vi "InfoRead4.vi"(4 "data info template":refnum<vi>, 5 "source path":string) -> (2 "data from *.info.txt":T1)   [LabVIEW 2014]
uses:
  <vilib>/Utility/file.llb/Read From Spreadsheet File (string).vi
panel:
  # "0 - aplly *.info.txt\n1 - Continue and enter the data manually\n2 - Cancel and correct the *.info.txt"
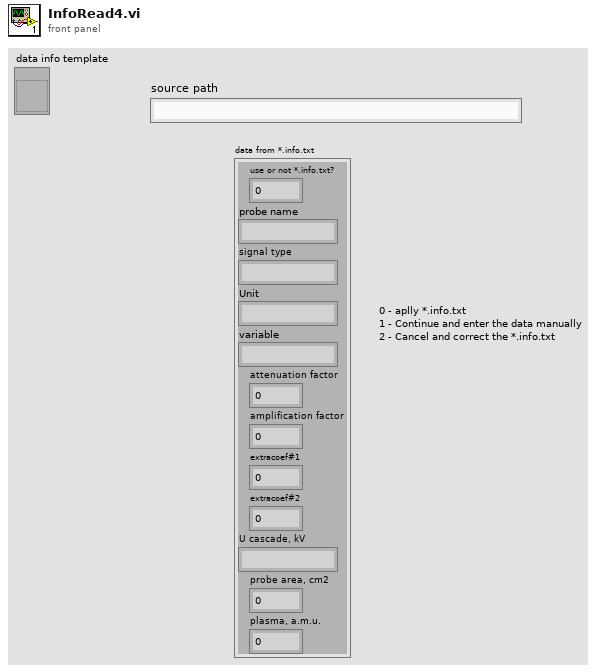
[diagram p1: front panel]
types:
  T1 = cluster{"use or not *.info.txt?":i16, "probe name":string, "signal type":string, "Unit":string, "variable":string, "attenuation factor":dbl, "amplification factor":dbl, "extracoef#1":dbl, "extracoef#2":dbl, "U cascade, kV":string, "probe area, cm2":dbl, "plasma, a.m.u.":dbl}
  T2 = cluster{"data path":string, "ADCintercadr_s":dbl, "data info":cluster{"use or not *.info.txt?":i16, "probe name":string, "signal type":string, "Unit":string, "variable":string, "attenuation factor":dbl, "amplification factor":dbl, "extracoef#1":dbl, "extracoef#2":dbl, "U cascade, kV":string, "probe area, cm2":dbl, "plasma, a.m.u.":dbl}, "channel_name":string, "channels_in_file":i32, "LastModified":string}
  T3 = enum16{"Left Button", "Center Button", "Right Button", "Window Close"}
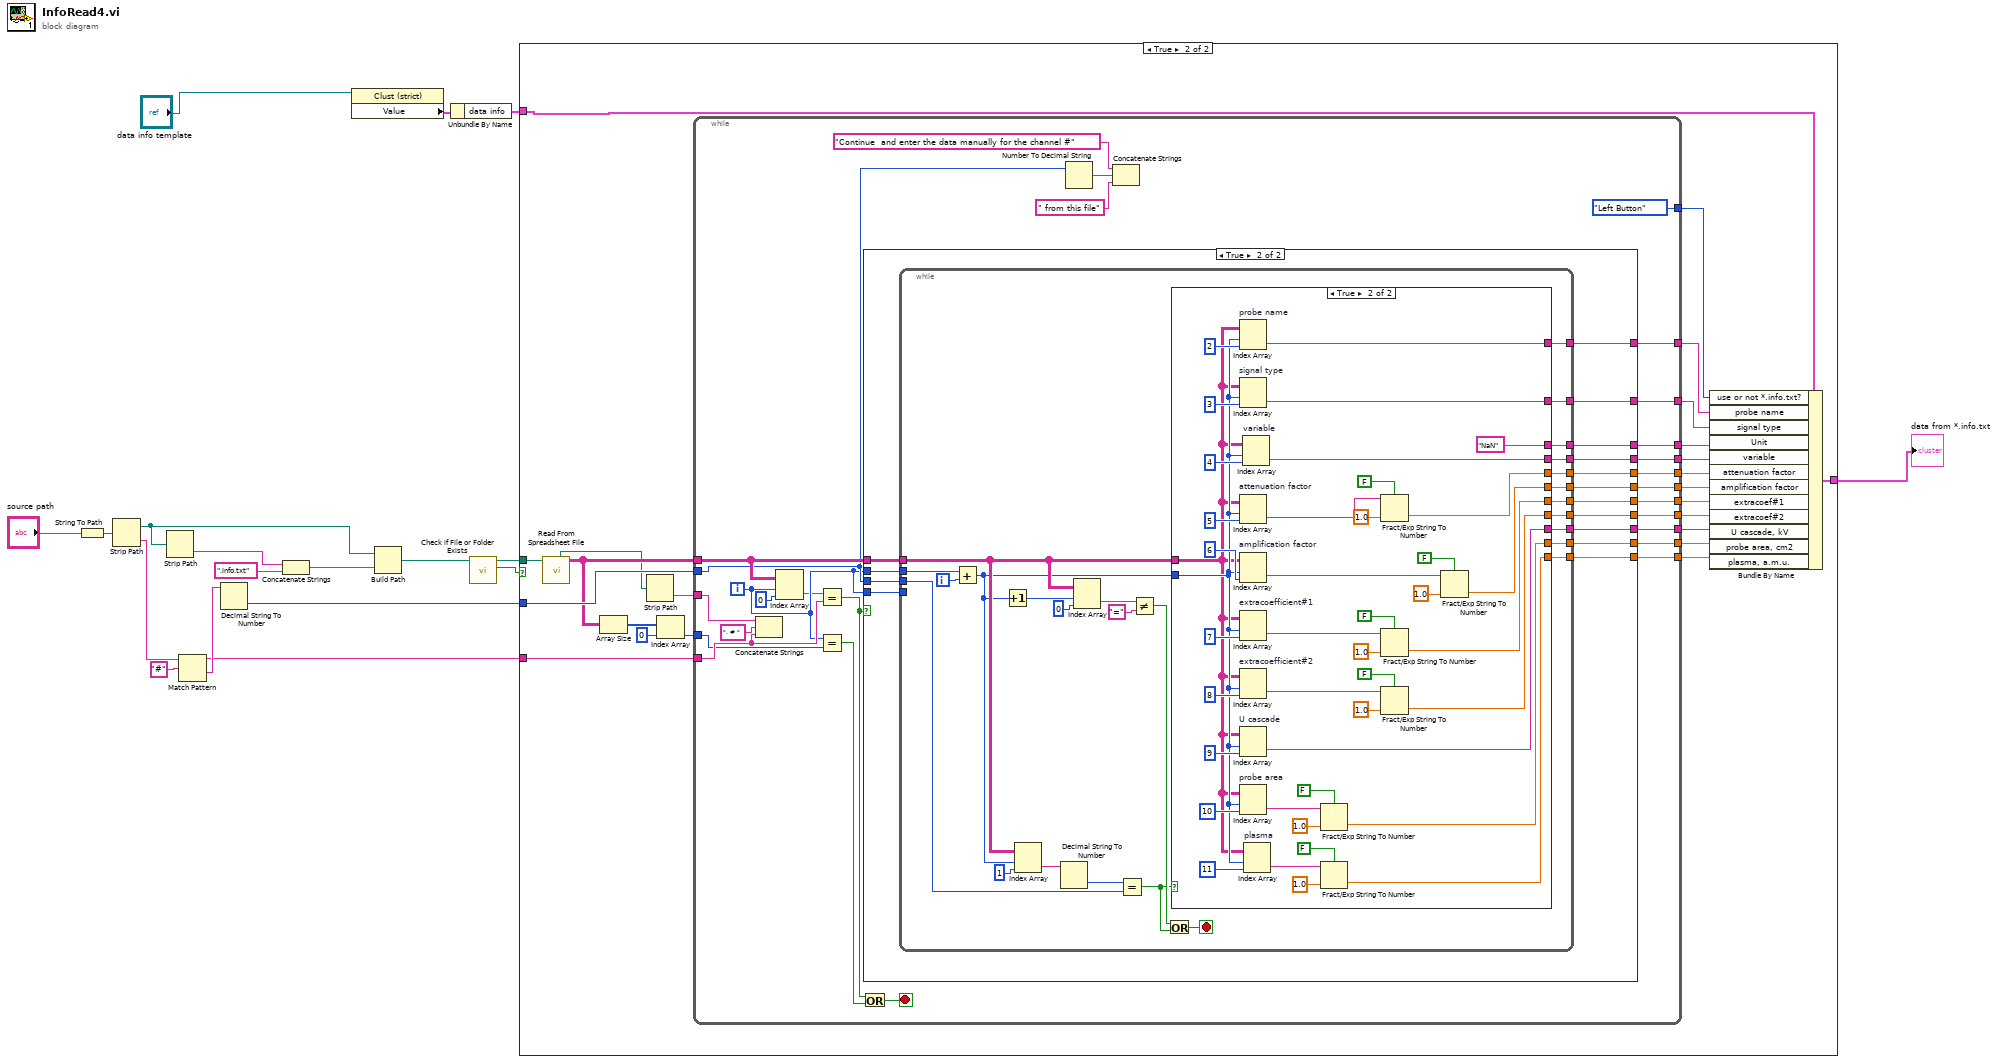
[diagram p0: block diagram]
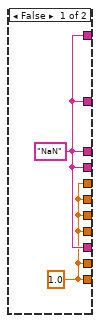
[diagram p3: hidden frame]
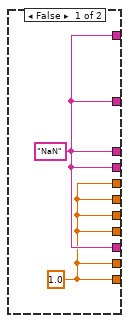
[diagram p4: hidden frame]
diagram:
  n1 = String To Path(string="source path") -> (path=w13:path)
  n2 = Strip Path(path=w13) -> (stripped path=w7:path, name=w17:string)
  n3 = Strip Path(path=w7) -> (name=w6:string)  [unwired: 1 out]
  n4 = Match Pattern(string=w17, regular expression="#") -> (before substring=w12:string, after substring=w15:string)  [unwired: 1 in, 2 out]
  n5 = Decimal String To Number(string=w15) -> (number=w14:i32)  [unwired: 2 in, 1 out]
  n6 = Concatenate Strings(w6, ".info.txt" ("string")) -> (w10:string)
  n7 = property class="Clust (strict)"(reference="data info template") -> ("Value"=w4:T2)  [unwired: 1 in, 2 out]
  n8 = Build Path(base path=w7, name or relative path=w10) -> (appended path=w9:path)
  n9 = Unbundle By Name(w4) -> ("data info"=w3:T1)
  n10 = call <vilib>:"Check if File or Folder Exists.vi"("path"=w9) -> ("file or folder exists?"=w5:bool, "dup path"=w8:path)  [unwired: 8 in, 1 out]
  n11 = case shown="True" w5 {
    tunnel: w14 -> [_ w39]
    tunnel: w12 -> [_ w38]
    tunnel: w8 -> [_ w36]
    tunnel: [w19 w20] -> w2
    tunnel: w3 -> [w19 w21]
    frame False {
    }
    frame True {
      n12 = call-poly <vilib>:"Read From Spreadsheet File.vi"("file path (dialog if empty)"=w36) -> ("all rows"=w37:string[][], "new file path (Not A Path if cancelled)"=w35:path)  [unwired: 6 in, 3 out]
      n13 = Array Size(array=w37) -> (size(s)=w41:i32[])
      n14 = Strip Path(path=w35) -> (name=w40:string)  [unwired: 1 out]
      n15 = Index Array(array=w41, index=0) -> (element=w34:i32)
      n16 = while {
        tunnel: w37 -> [w65]
        tunnel: [T3."Left Button" ("Which Button?")] -> w33
        tunnel: w39 -> [w59]
        tunnel: w40 -> [w61]
        tunnel: w38 -> [w58]
        tunnel: w34 -> [w57]
        tunnel: [w56] -> w32
        tunnel: [w55] -> w31
        tunnel: [w54] -> w30
        tunnel: [w53] -> w29
        tunnel: [w52] -> w28
        tunnel: [w51] -> w27
        tunnel: [w50] -> w26
        tunnel: [w49] -> w25
        tunnel: [w48] -> w24
        tunnel: [w47] -> w23
        tunnel: [w46] -> w22
        i -> [w45]
        stop <- w68 stop-if-true
        n17 = Concatenate Strings(w61, ", # " ("string"), w58) -> ()  [unwired: 1 out]
        n18 = Index Array(array=w65, index (row)=w45, index (col)=0 ("disabled index (col)")) -> (element=w44:string)
        n19 = Equal?(x=w44, y=w58) -> (x = y?=w66:bool)
        n20 = Equal?(x=w45, y=w57) -> (x = y?=w67:bool)
        n21 = Or(x=w66, y=w67) -> (x .or. y?=w68:bool)
        n22 = case shown="True" w66 {
          tunnel: w65 -> [_ w73]
          tunnel: w59 -> [_ w86]
          tunnel: w45 -> [_ w85]
          tunnel: [w71 w83] -> w56
          tunnel: [w71 w82] -> w55
          tunnel: [w71 w84] -> w54
          tunnel: [w71 w81] -> w53
          tunnel: [w71 w76] -> w52
          tunnel: [w70 w80] -> w51
          tunnel: [w70 w79] -> w50
          tunnel: [w70 w78] -> w49
          tunnel: [w70 w77] -> w48
          tunnel: [w70 w75] -> w47
          tunnel: [w70 w74] -> w46
          tunnel: w45 -> [_ w72]
          frame False {
            w70 = 1.0
            w71 = "NaN" ("String")
          }
          frame True {
            n23 = while {
              tunnel: w86 -> [w112]
              tunnel: w85 -> [_]
              tunnel: [w111] -> w84
              tunnel: [w110] -> w83
              tunnel: [w109] -> w82
              tunnel: [w108] -> w81
              tunnel: [w107] -> w80
              tunnel: [w106] -> w79
              tunnel: [w105] -> w78
              tunnel: [w104] -> w77
              tunnel: [w103] -> w76
              tunnel: [w102] -> w75
              tunnel: [w101] -> w74
              tunnel: w73 -> [w94]
              tunnel: w72 -> [w98]
              i -> [w97]
              stop <- w89 stop-if-true
              n24 = Add(x=w98, y=w97) -> (x+y=w90:i32)
              n25 = Increment(x=w90) -> (x+1=w91:i32)
              n26 = Index Array(array=w94, index (row)=w90, index (col)=1 ("disabled index (col)")) -> (element=w99:string)
              n27 = Decimal String To Number(string=w99) -> (number=w100:i32)  [unwired: 2 in, 1 out]
              n28 = Index Array(array=w94, index (row)=w91, index (col)=0 ("disabled index (col)")) -> (element=w93:string)
              n29 = Equal?(x=w100, y=w112) -> (x = y?=w87:bool)
              n30 = Not Equal?(x=w93, y="=") -> (x != y?=w88:bool)
              n31 = Or(x=w88, y=w87) -> (x .or. y?=w89:bool)
              n32 = case shown="True" w87 {
                tunnel: [w114 "NaN"] -> w111
                tunnel: [w114 w130] -> w110
                tunnel: [w114 w129] -> w109
                tunnel: [w114 w128] -> w108
                tunnel: [w113 w127] -> w107
                tunnel: [w113 w126] -> w106
                tunnel: [w113 w125] -> w105
                tunnel: w90 -> [_ w123]
                tunnel: [w113 w119] -> w104
                tunnel: [w114 w118] -> w103
                tunnel: [w113 w117] -> w102
                tunnel: [w113 w116] -> w101
                tunnel: w94 -> [_ w115]
                frame False {
                  w113 = 1.0
                  w114 = "NaN"
                }
                frame True {
                  n33 = Index Array "probe name"(array=w115, index (row)=w123, index (col)=2 ("disabled index (col)")) -> (element=w130:string)
                  n34 = Index Array "signal type"(array=w115, index (row)=w123, index (col)=3 ("disabled index (col)")) -> (element=w129:string)
                  n35 = Index Array "attenuation factor"(array=w115, index (row)=w123, index (col)=5 ("disabled index (col)")) -> (element=w140:string)
                  n36 = Index Array "amplification factor"(array=w115, index (row)=w123, index (col)=6 ("disabled index (col)")) -> (element=w141:string)
                  n37 = Index Array "extracoefficient#1"(array=w115, index (row)=w123, index (col)=7 ("disabled index (col)")) -> (element=w148:string)
                  n38 = Index Array "extracoefficient#2"(array=w115, index (row)=w123, index (col)=8 ("disabled index (col)")) -> (element=w120:string)
                  n39 = Index Array "U cascade"(array=w115, index (row)=w123, index (col)=9 ("disabled index (col)")) -> (element=w118:string)
                  n40 = Index Array "probe area"(array=w115, index (row)=w123, index (col)=10 ("disabled index (col)")) -> (element=w136:string)
                  n41 = Index Array "variable"(array=w115, index (row)=w123, index (col)=4 ("disabled index (col)")) -> (element=w128:string)
                  n42 = Index Array "plasma"(array=w115, index (row)=w123, index (col)=11 ("disabled index (col)")) -> (element=w132:string)
                  n43 = Fract/Exp String To Number(use system decimal point (T)=FALSE, string=w136, default (0 dbl)=1.0 ("default (0 DBL)")) -> (number=w117:dbl)  [unwired: 1 in, 1 out]
                  n44 = Fract/Exp String To Number(use system decimal point (T)=FALSE, string=w132, default (0 dbl)=1.0 ("default (0 DBL)")) -> (number=w116:dbl)  [unwired: 1 in, 1 out]
                  n45 = Fract/Exp String To Number(use system decimal point (T)=FALSE, string=w140, default (0 dbl)=1.0 ("default (0 DBL)")) -> (number=w127:dbl)  [unwired: 1 in, 1 out]
                  n46 = Fract/Exp String To Number(use system decimal point (T)=FALSE, string=w148, default (0 dbl)=1.0 ("default (0 DBL)")) -> (number=w125:dbl)  [unwired: 1 in, 1 out]
                  n47 = Fract/Exp String To Number(use system decimal point (T)=FALSE, string=w120, default (0 dbl)=1.0 ("default (0 DBL)")) -> (number=w119:dbl)  [unwired: 1 in, 1 out]
                  n48 = Fract/Exp String To Number(use system decimal point (T)=FALSE, string=w141, default (0 dbl)=1.0 ("default (0 DBL)")) -> (number=w126:dbl)  [unwired: 1 in, 1 out]
                }
              }
            }
          }
        }
        n49 = Number To Decimal String(number=w59) -> (decimal integer string=w63:string)  [unwired: 1 in]
        n50 = Concatenate Strings("Continue  and enter the data manually for the channel #" ("Left Button Text (\"Yes\")"), w63, " from this file" ("string")) -> ()  [unwired: 1 out]
      }
      n51 = Bundle By Name(cluster=w21, "use or not *.info.txt?"=w33, "probe name"=w32, "signal type"=w31, "Unit"=w30, "variable"=w29, "attenuation factor"=w27, "amplification factor"=w26, "extracoef#1"=w25, "extracoef#2"=w24, "U cascade, kV"=w28, "probe area, cm2"=w23, "plasma, a.m.u."=w22) -> (w20:T1)
    }
  }
  "data from *.info.txt" <- w2
